vi "Clean and Get Names.vi"(8 "error in":errorcluster, 11 "Working Dir":path) -> (0 "error out":errorcluster, 1 "Deleted files":string[](array[string]), 2 "filenames":string[](array[string]), 3 "Working Dir Out":path)   [LabVIEW 2024]
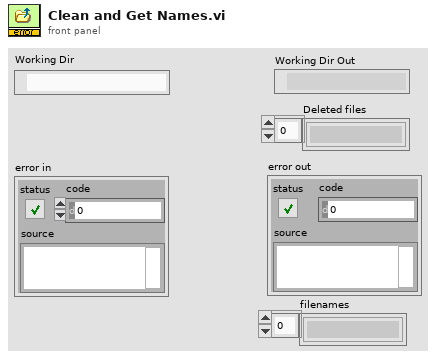
[diagram p1: front panel]
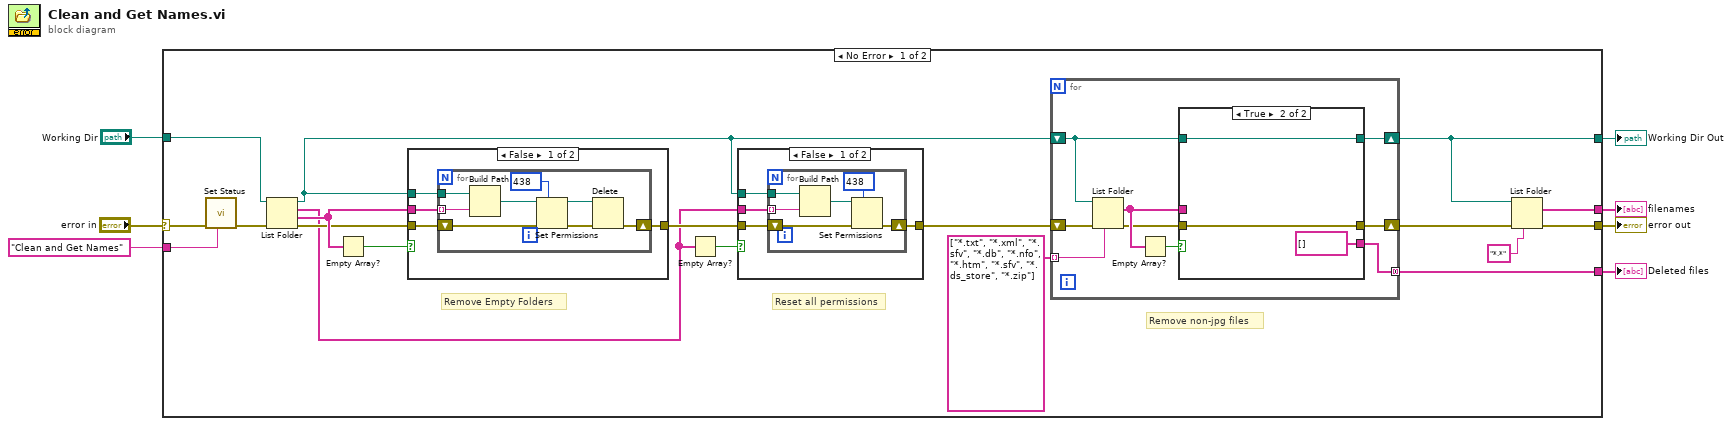
[diagram p0: block diagram]
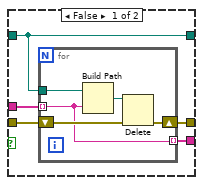
[diagram p3: hidden frame]
diagram:
  n1 = case shown="No Error" "error in" {
    selector: "error in" -> [w15 w73]
    tunnel: "Working Dir" -> [w23 w74]
    tunnel: [w20 w74] -> w6
    tunnel: [w19 w73] -> w5
    tunnel: [w18 _] -> w4
    tunnel: [w17 _] -> w3
    tunnel: "Clean and Get Names" ("Value") -> [w13 _]
    frame No Error {
      # "Reset all permissions"
      # "Remove non-jpg files"
      # "Remove Empty Folders"
      n2 = call "Set Status.vi"("Status Message"=w13, "error in (no error)"=w15) -> ("error out"=w14:errorcluster)  [unwired: 9 in]
      n3 = List Folder(path=w23, error in=w14) -> (path out=w11:path, filenames=w8:string[], folder names=w25:string[], error out=w24:errorcluster)  [unwired: 2 in]
      n4 = Empty Array?(array=w25) -> (empty?=w26:bool)
      n5 = case shown="False" w26 {
        tunnel: w25 -> [w63 _]
        tunnel: w11 -> [w60 _]
        tunnel: w24 -> [w62 w72]
        tunnel: [w61 w72] -> w12
        frame False {
          n6 = for {
            tunnel: w63 -> [w70] mode=indexing
            tunnel: w60 -> [w71]
            shift-right: [w69] -> w61
            shift-left: w62 -> [w64]
            n7 = Build Path(base path=w71, name or relative path=w70) -> (appended path=w65:path)
            n8 = Set Permissions(7:i16 438 ("permissions"), 8:w64, 11:w65) -> (0:w68:errorcluster, 3:w67:path)  [unwired: 2 in]
            n9 = Delete(path (use dialog)=w67, error in=w68) -> (error out=w69:errorcluster)  [unwired: 3 in, 2 out]
          }
        }
        frame True {
        }
      }
      n10 = Empty Array?(array=w8) -> (empty?=w9:bool)
      n11 = case shown="False" w9 {
        tunnel: w8 -> [w30 _]
        tunnel: w11 -> [w27 _]
        tunnel: w12 -> [w29 w37]
        tunnel: [w28 w37] -> w10
        frame False {
          n12 = for {
            tunnel: w30 -> [w35] mode=indexing
            tunnel: w27 -> [w36]
            shift-right: [w32] -> w28
            shift-left: w29 -> [w33]
            n13 = Build Path(base path=w36, name or relative path=w35) -> (appended path=w31:path)
            n14 = Set Permissions(7:i16 438 ("permissions"), 8:w33, 11:w31) -> (0:w32:errorcluster)  [unwired: 2 in, 1 out]
          }
        }
        frame True {
        }
      }
      n15 = for {
        shift-right: [w40] -> w21
        shift-left: w10 -> [w46]
        tunnel: string[] ["*.txt", "*.xml", "*.sfv", "*.db", "*.nfo", "*.htm", "*.sfv", "*.ds_store", "*.zip"] -> [w45] mode=indexing
        shift-right: [w39] -> w20
        shift-left: w11 -> [w44]
        tunnel: [w38] -> w18 mode=concatenating
        n16 = List Folder(path=w44, pattern=w45, error in=w46) -> (filenames=w42:string[], error out=w41:errorcluster)  [unwired: 1 in, 2 out]
        n17 = Empty Array?(array=w42) -> (empty?=w43:bool)
        n18 = case shown="True" w43 {
          tunnel: w42 -> [w51 _]
          tunnel: w44 -> [w48 w58]
          tunnel: w41 -> [w50 w59]
          tunnel: [w49 w59] -> w40
          tunnel: [w48 w58] -> w39
          tunnel: [w47 string[] []] -> w38
          frame False {
            n19 = for {
              tunnel: w51 -> [w52] mode=indexing
              tunnel: w48 -> [w55]
              shift-right: [w53] -> w49
              shift-left: w50 -> [w54]
              tunnel: [w52] -> w47 mode=indexing
              n20 = Build Path(base path=w55, name or relative path=w52) -> (appended path=w56:path)
              n21 = Delete(path (use dialog)=w56, error in=w54) -> (error out=w53:errorcluster)  [unwired: 3 in, 2 out]
            }
          }
          frame True {
          }
        }
      }
      n22 = List Folder(path=w20, pattern="*.*", error in=w21) -> (filenames=w17:string[], error out=w19:errorcluster)  [unwired: 1 in, 2 out]
    }
    frame Error {
    }
  }
  "Working Dir Out" <- w6
  "error out" <- w5
  "Deleted files" <- w4
  "filenames" <- w3
